vi "TalonFXSGetters.vi"   [LabVIEW 2025]
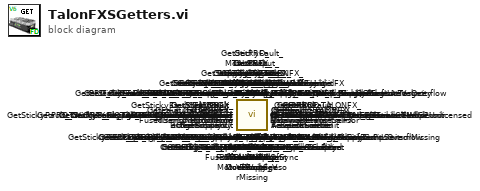
[diagram p0: block diagram]
diagram:
  n1 = call <vilib>:"GetStickyFault_TALONFX_5V.vi"() -> ()  [unwired: 10 in, 2 out]
  n2 = call <vilib>:"GetFault_TALONFX_5V.vi"() -> ()  [unwired: 10 in, 2 out]
  n3 = call <vilib>:"GetStickyFault_TALONFX_MotorArrangementNotSelected.vi"() -> ()  [unwired: 10 in, 2 out]
  n4 = call <vilib>:"GetFault_TALONFX_MotorArrangementNotSelected.vi"() -> ()  [unwired: 10 in, 2 out]
  n5 = call <vilib>:"GetStickyFault_TALONFX_MotorTempSensorTooHot.vi"() -> ()  [unwired: 10 in, 2 out]
  n6 = call <vilib>:"GetFault_TALONFX_MotorTempSensorTooHot.vi"() -> ()  [unwired: 10 in, 2 out]
  n7 = call <vilib>:"GetStickyFault_TALONFX_MotorTempSensorMissing.vi"() -> ()  [unwired: 10 in, 2 out]
  n8 = call <vilib>:"GetFault_TALONFX_MotorTempSensorMissing.vi"() -> ()  [unwired: 10 in, 2 out]
  n9 = call <vilib>:"GetStickyFault_TALONFX_DriveDisabledHallSensor.vi"() -> ()  [unwired: 10 in, 2 out]
  n10 = call <vilib>:"GetFault_TALONFX_DriveDisabledHallSensor.vi"() -> ()  [unwired: 10 in, 2 out]
  n11 = call <vilib>:"GetStickyFault_TALONFX_HallSensorMissing.vi"() -> ()  [unwired: 10 in, 2 out]
  n12 = call <vilib>:"GetFault_TALONFX_HallSensorMissing.vi"() -> ()  [unwired: 10 in, 2 out]
  n13 = call <vilib>:"GetStickyFault_TALONFX_BridgeShort.vi"() -> ()  [unwired: 10 in, 2 out]
  n14 = call <vilib>:"GetFault_TALONFX_BridgeShort.vi"() -> ()  [unwired: 10 in, 2 out]
  n15 = call <vilib>:"GetStickyFault_TALONFX_StaticBrakeDisabled.vi"() -> ()  [unwired: 10 in, 2 out]
  n16 = call <vilib>:"GetFault_TALONFX_StaticBrakeDisabled.vi"() -> ()  [unwired: 10 in, 2 out]
  n17 = call <vilib>:"GetStickyFault_TALONFX_UsingFusedCCWhileUnlicensed.vi"() -> ()  [unwired: 10 in, 2 out]
  n18 = call <vilib>:"GetFault_TALONFX_UsingFusedCCWhileUnlicensed.vi"() -> ()  [unwired: 10 in, 2 out]
  n19 = call <vilib>:"GetStickyFault_TALONFX_SupplyCurrLimit.vi"() -> ()  [unwired: 10 in, 2 out]
  n20 = call <vilib>:"GetFault_TALONFX_SupplyCurrLimit.vi"() -> ()  [unwired: 10 in, 2 out]
  n21 = call <vilib>:"GetStickyFault_TALONFX_StatorCurrLimit.vi"() -> ()  [unwired: 10 in, 2 out]
  n22 = call <vilib>:"GetFault_TALONFX_StatorCurrLimit.vi"() -> ()  [unwired: 10 in, 2 out]
  n23 = call <vilib>:"GetStickyFault_TALONFX_FusedSensorOutOfSync.vi"() -> ()  [unwired: 10 in, 2 out]
  n24 = call <vilib>:"GetFault_TALONFX_FusedSensorOutOfSync.vi"() -> ()  [unwired: 10 in, 2 out]
  n25 = call <vilib>:"GetStickyFault_TALONFX_MissingRemoteSensor.vi"() -> ()  [unwired: 10 in, 2 out]
  n26 = call <vilib>:"GetFault_TALONFX_MissingRemoteSensor.vi"() -> ()  [unwired: 10 in, 2 out]
  n27 = call <vilib>:"GetStickyFault_TALONFX_MissingRemHardLim.vi"() -> ()  [unwired: 10 in, 2 out]
  n28 = call <vilib>:"GetFault_TALONFX_MissingRemHardLim.vi"() -> ()  [unwired: 10 in, 2 out]
  n29 = call <vilib>:"GetStickyFault_TALONFX_MissingRemSoftLim.vi"() -> ()  [unwired: 10 in, 2 out]
  n30 = call <vilib>:"GetFault_TALONFX_MissingRemSoftLim.vi"() -> ()  [unwired: 10 in, 2 out]
  n31 = call <vilib>:"GetStickyFault_TALONFX_ForwardSoftLimit.vi"() -> ()  [unwired: 10 in, 2 out]
  n32 = call <vilib>:"GetFault_TALONFX_ForwardSoftLimit.vi"() -> ()  [unwired: 10 in, 2 out]
  n33 = call <vilib>:"GetStickyFault_TALONFX_ReverseSoftLimit.vi"() -> ()  [unwired: 10 in, 2 out]
  n34 = call <vilib>:"GetFault_TALONFX_ReverseSoftLimit.vi"() -> ()  [unwired: 10 in, 2 out]
  n35 = call <vilib>:"GetStickyFault_TALONFX_ForwardHardLimit.vi"() -> ()  [unwired: 10 in, 2 out]
  n36 = call <vilib>:"GetFault_TALONFX_ForwardHardLimit.vi"() -> ()  [unwired: 10 in, 2 out]
  n37 = call <vilib>:"GetStickyFault_TALONFX_ReverseHardLimit.vi"() -> ()  [unwired: 10 in, 2 out]
  n38 = call <vilib>:"GetFault_TALONFX_ReverseHardLimit.vi"() -> ()  [unwired: 10 in, 2 out]
  n39 = call <vilib>:"GetStickyFault_TALONFX_UnstableSupplyV.vi"() -> ()  [unwired: 10 in, 2 out]
  n40 = call <vilib>:"GetFault_TALONFX_UnstableSupplyV.vi"() -> ()  [unwired: 10 in, 2 out]
  n41 = call <vilib>:"GetStickyFault_TALONFX_OverSupplyV.vi"() -> ()  [unwired: 10 in, 2 out]
  n42 = call <vilib>:"GetFault_TALONFX_OverSupplyV.vi"() -> ()  [unwired: 10 in, 2 out]
  n43 = call <vilib>:"GetStickyFault_TALONFX_RemoteSensorPosOverflow.vi"() -> ()  [unwired: 10 in, 2 out]
  n44 = call <vilib>:"GetFault_TALONFX_RemoteSensorPosOverflow.vi"() -> ()  [unwired: 10 in, 2 out]
  n45 = call <vilib>:"GetStickyFault_TALONFX_MissingDifferentialFX.vi"() -> ()  [unwired: 10 in, 2 out]
  n46 = call <vilib>:"GetFault_TALONFX_MissingDifferentialFX.vi"() -> ()  [unwired: 10 in, 2 out]
  n47 = call <vilib>:"GetStickyFault_TALONFX_RemoteSensorReset.vi"() -> ()  [unwired: 10 in, 2 out]
  n48 = call <vilib>:"GetFault_TALONFX_RemoteSensorReset.vi"() -> ()  [unwired: 10 in, 2 out]
  n49 = call <vilib>:"GetStickyFault_TALONFX_BridgeBrownout.vi"() -> ()  [unwired: 10 in, 2 out]
  n50 = call <vilib>:"GetFault_TALONFX_BridgeBrownout.vi"() -> ()  [unwired: 10 in, 2 out]
  n51 = call <vilib>:"GetStickyFault_UnlicensedFeatureInUse.vi"() -> ()  [unwired: 10 in, 2 out]
  n52 = call <vilib>:"GetFault_UnlicensedFeatureInUse.vi"() -> ()  [unwired: 10 in, 2 out]
  n53 = call <vilib>:"GetStickyFault_BootDuringEnable.vi"() -> ()  [unwired: 10 in, 2 out]
  n54 = call <vilib>:"GetFault_BootDuringEnable.vi"() -> ()  [unwired: 10 in, 2 out]
  n55 = call <vilib>:"GetStickyFault_Undervoltage.vi"() -> ()  [unwired: 10 in, 2 out]
  n56 = call <vilib>:"GetFault_Undervoltage.vi"() -> ()  [unwired: 10 in, 2 out]
  n57 = call <vilib>:"GetStickyFault_DeviceTemp.vi"() -> ()  [unwired: 10 in, 2 out]
  n58 = call <vilib>:"GetFault_DeviceTemp.vi"() -> ()  [unwired: 10 in, 2 out]
  n59 = call <vilib>:"GetStickyFault_ProcTemp.vi"() -> ()  [unwired: 10 in, 2 out]
  n60 = call <vilib>:"GetFault_ProcTemp.vi"() -> ()  [unwired: 10 in, 2 out]
  n61 = call <vilib>:"GetStickyFault_Hardware.vi"() -> ()  [unwired: 10 in, 2 out]
  n62 = call <vilib>:"GetFault_Hardware.vi"() -> ()  [unwired: 10 in, 2 out]
  n63 = call <vilib>:"GetPRO_GadgeteerPwm_RawPwmVelocity.vi"() -> ()  [unwired: 10 in, 2 out]
  n64 = call <vilib>:"GetPRO_GadgeteerPwm_RawPwmPosition.vi"() -> ()  [unwired: 10 in, 2 out]
  n65 = call <vilib>:"GetPRO_GadgeteerQuad_RawQuadratureVelocity.vi"() -> ()  [unwired: 10 in, 2 out]
  n66 = call <vilib>:"GetPRO_GadgeteerQuad_RawQuadraturePosition.vi"() -> ()  [unwired: 10 in, 2 out]
  n67 = call <vilib>:"GetTalonFXS_Gadgeteer_G3.vi"() -> ()  [unwired: 10 in, 2 out]
  n68 = call <vilib>:"GetTalonFXS_5VRailVoltage.vi"() -> ()  [unwired: 10 in, 2 out]
  n69 = call <vilib>:"GetTalonFX_ConnectedMotor.vi"() -> ()  [unwired: 10 in, 2 out]
  n70 = call <vilib>:"GetPRO_SupplyAndTemp_DeviceTemp2.vi"() -> ()  [unwired: 10 in, 2 out]
  n71 = call <vilib>:"GetVersion_IsProLicensed.vi"() -> ()  [unwired: 10 in, 2 out]
  n72 = call <vilib>:"GetPRO_MotorOutput_BridgeType_Public.vi"() -> ()  [unwired: 10 in, 2 out]
  n73 = call <vilib>:"GetTalonFX_MotorConstants_StallCurrent.vi"() -> ()  [unwired: 10 in, 2 out]
  n74 = call <vilib>:"GetTalonFX_MotorConstants_kV.vi"() -> ()  [unwired: 10 in, 2 out]
  n75 = call <vilib>:"GetTalonFX_MotorConstants_kT.vi"() -> ()  [unwired: 10 in, 2 out]
  n76 = call <vilib>:"GetPRO_DiffPIDOutput_Slot.vi"() -> ()  [unwired: 10 in, 2 out]
  n77 = call <vilib>:"GetPRO_DiffPosAndVel_Position.vi"() -> ()  [unwired: 10 in, 2 out]
  n78 = call <vilib>:"GetPRO_DiffPosAndVel_Velocity.vi"() -> ()  [unwired: 10 in, 2 out]
  n79 = call <vilib>:"GetPRO_AvgPosAndVel_Position.vi"() -> ()  [unwired: 10 in, 2 out]
  n80 = call <vilib>:"GetPRO_AvgPosAndVel_Velocity.vi"() -> ()  [unwired: 10 in, 2 out]
  n81 = call <vilib>:"GetTalonFX_DifferentialControlMode.vi"() -> ()  [unwired: 10 in, 2 out]
  n82 = call <vilib>:"GetTalonFX_MotorOutputStatus.vi"() -> ()  [unwired: 10 in, 2 out]
  n83 = call <vilib>:"GetPRO_PIDOutput_Slot.vi"() -> ()  [unwired: 10 in, 2 out]
  n84 = call <vilib>:"GetPRO_PIDStateEnables_DeviceEnable.vi"() -> ()  [unwired: 10 in, 2 out]
  n85 = call <vilib>:"GetPRO_PIDStateEnables_RobotEnable.vi"() -> ()  [unwired: 10 in, 2 out]
  n86 = call <vilib>:"GetPRO_PIDStateEnables_IsMotionMagicRunning.vi"() -> ()  [unwired: 10 in, 2 out]
  n87 = call <vilib>:"GetPRO_PIDStateEnables_MotionMagicAtTarget.vi"() -> ()  [unwired: 10 in, 2 out]
  n88 = call <vilib>:"GetExternalMotorTemp.vi"() -> ()  [unwired: 10 in, 2 out]
  n89 = call <vilib>:"GetExternalMotorTempStatus.vi"() -> ()  [unwired: 10 in, 2 out]
  n90 = call <vilib>:"GetTalonFX_ControlMode.vi"() -> ()  [unwired: 10 in, 2 out]
  n91 = call <vilib>:"GetPRO_PosAndVel_Acceleration.vi"() -> ()  [unwired: 10 in, 2 out]
  n92 = call <vilib>:"GetPRO_PosAndVel_Position.vi"() -> ()  [unwired: 10 in, 2 out]
  n93 = call <vilib>:"GetPRO_PosAndVel_Velocity.vi"() -> ()  [unwired: 10 in, 2 out]
  n94 = call <vilib>:"GetPRO_RotorPosAndVel_Position.vi"() -> ()  [unwired: 10 in, 2 out]
  n95 = call <vilib>:"GetPRO_RotorPosAndVel_Velocity.vi"() -> ()  [unwired: 10 in, 2 out]
  n96 = call <vilib>:"GetPRO_SupplyAndTemp_ProcessorTemp.vi"() -> ()  [unwired: 10 in, 2 out]
  n97 = call <vilib>:"GetPRO_SupplyAndTemp_DeviceTemp.vi"() -> ()  [unwired: 10 in, 2 out]
  n98 = call <vilib>:"GetPRO_SupplyAndTemp_SupplyVoltage.vi"() -> ()  [unwired: 10 in, 2 out]
  n99 = call <vilib>:"GetPRO_SupplyAndTemp_SupplyCurrent.vi"() -> ()  [unwired: 10 in, 2 out]
  n100 = call <vilib>:"GetPRO_SupplyAndTemp_StatorCurrent.vi"() -> ()  [unwired: 10 in, 2 out]
  n101 = call <vilib>:"GetPRO_MotorOutput_TorqueCurrent.vi"() -> ()  [unwired: 10 in, 2 out]
  n102 = call <vilib>:"GetPRO_MotorOutput_DutyCycle.vi"() -> ()  [unwired: 10 in, 2 out]
  n103 = call <vilib>:"GetPRO_MotorOutput_RotorPolarity.vi"() -> ()  [unwired: 10 in, 2 out]
  n104 = call <vilib>:"GetReverseLimit.vi"() -> ()  [unwired: 10 in, 2 out]
  n105 = call <vilib>:"GetForwardLimit.vi"() -> ()  [unwired: 10 in, 2 out]
  n106 = call <vilib>:"GetPRO_MotorOutput_MotorVoltage.vi"() -> ()  [unwired: 10 in, 2 out]
  n107 = call <vilib>:"GetAllStickyFaults.vi"() -> ()  [unwired: 10 in, 2 out]
  n108 = call <vilib>:"GetAllFaults.vi"() -> ()  [unwired: 10 in, 2 out]
  n109 = call <vilib>:"GetVersion_Full.vi"() -> ()  [unwired: 10 in, 2 out]
  n110 = call <vilib>:"GetVersion_Build.vi"() -> ()  [unwired: 10 in, 2 out]
  n111 = call <vilib>:"GetVersion_Bugfix.vi"() -> ()  [unwired: 10 in, 2 out]
  n112 = call <vilib>:"GetVersion_Minor.vi"() -> ()  [unwired: 10 in, 2 out]
  n113 = call <vilib>:"GetVersion_Major.vi"() -> ()  [unwired: 10 in, 2 out]
